vi "Do.vi"(8 "error in":errorcluster, 10 "Actor in":refnum<class "Actor.lvclass">, 11 "Change File MSG":refnum<class "Change File MSG.lvclass">) -> (0 "error out":errorcluster, 2 "Actor out":refnum<class "Actor.lvclass">)   [LabVIEW 2014, in "File Library.lvlib" / "Change File MSG.lvclass"]
doc: "(<B>Filename</B>: Actor Framework.lvlib:Message.lvclass:Do.vi)\n\nDefines what a message does when it is received by an actor. Generally, a message instructs an actor to invoke one of its methods. By default, this method does nothing. A child class must override it to define behavior. Create a child class by using the Actor Framework Message Maker dialog box."
uses:
  Change File MSG.lvclass
  <vilib>/ActorFramework/Actor/Actor.lvclass
  File Actor.lvclass
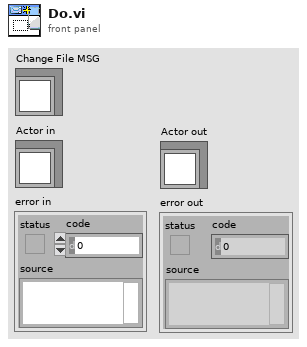
[diagram p1: front panel]
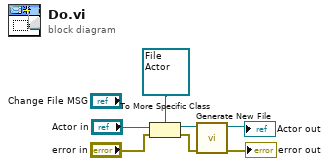
[diagram p0: block diagram]
diagram:
  n1 = To More Specific Class(target class=refnum<class "File Actor.lvclass"> refnum ("File Library.lvlib:File Actor"), reference="Actor in", error in="error in") -> (specific class reference=w5:refnum<class "File Actor.lvclass">, error out=w4:errorcluster)
  n2 = call "Generate New File.vi"("error in"=w4, "File Actor in"=w5) -> ("error out"=→"error out":errorcluster, "File Actor out"=→"Actor out":refnum<class "File Actor.lvclass">)  [unwired: 8 in]
